vi "FlatToRichhwval_GenericRequest.vi"(5 "OutputClusterType":T1, 11 "InputCluster":T3) -> (3 "OutputCluster":T1)   [LabVIEW 2025, in "ExamplePluginOOBService_client.lvlib"]
uses:
  hwval_GenericRequest_Flat.ctl
  google_protobuf_Any_Flat.ctl
  hwval_GenericRequest.ctl
  google_protobuf_Any.ctl
  ExamplePluginOOBService_client.lvlib
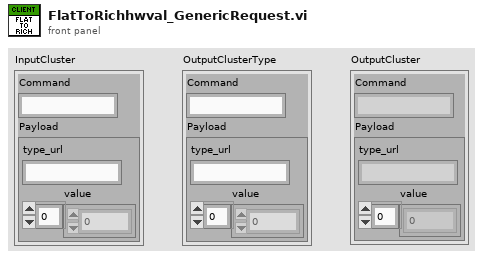
[diagram p1: front panel]
types:
  T1 = typedef "ExamplePluginOOBService_client.lvlib/hwval_GenericRequest.ctl" = cluster{"Command":string, "Payload":T2}
  T2 = typedef "ExamplePluginOOBService_client.lvlib/google_protobuf_Any.ctl" = cluster{"type_url":string, "value":u8[]}
  T3 = typedef "ExamplePluginOOBService_client.lvlib/hwval_GenericRequest_Flat.ctl" = cluster{"Command":string, "Payload":T4}
  T4 = typedef "ExamplePluginOOBService_client.lvlib/google_protobuf_Any_Flat.ctl" = cluster{"type_url":string, "value":u8[]}
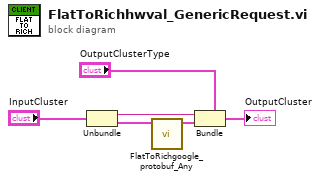
[diagram p0: block diagram]
diagram:
  n1 = Unbundle "Unbundle"("InputCluster") -> ("Command"=w3:string, "Payload"=w2:T4)
  n2 = call "FlatToRichgoogle_protobuf_Any.vi"("InputCluster"=w2) -> ("OutputCluster"=w1:T2)  [unwired: 10 in]
  n3 = Bundle "Bundle"(cluster="OutputClusterType", "Command"=w3, "Payload"=w1) -> (→"OutputCluster":T1)
